vi "Find Running VIs.vi"(8 "error in":errorcluster, 10 "Find Sub-VIs (T)":bool=TRUE, 11 "Find Top-Level VIs (T)":bool=TRUE) -> (0 "error out":errorcluster, 1 "New VIs Found":string[][](array[string]), 2 "#VIs Found":i32, 3 "VIs Found":string[][](array[string]), 4 "#New VIs Found":i32)   [LabVIEW 2022 SP3, in "hse-misc.lvlib"]
doc: "____\nHAMPEL SOFTWARE ENGINEERING v3.8.0 (2023-12-18 14:41)"
uses:
  hse-misc.lvlib
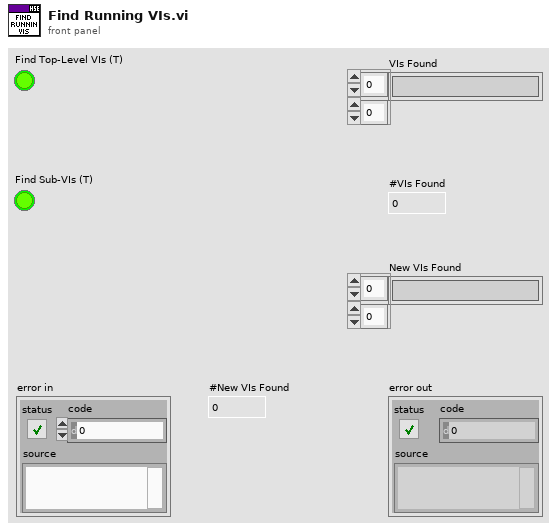
[diagram p1: front panel]
types:
  T1 = enum32{"Bad", "Idle", "Run top level", "Running"}
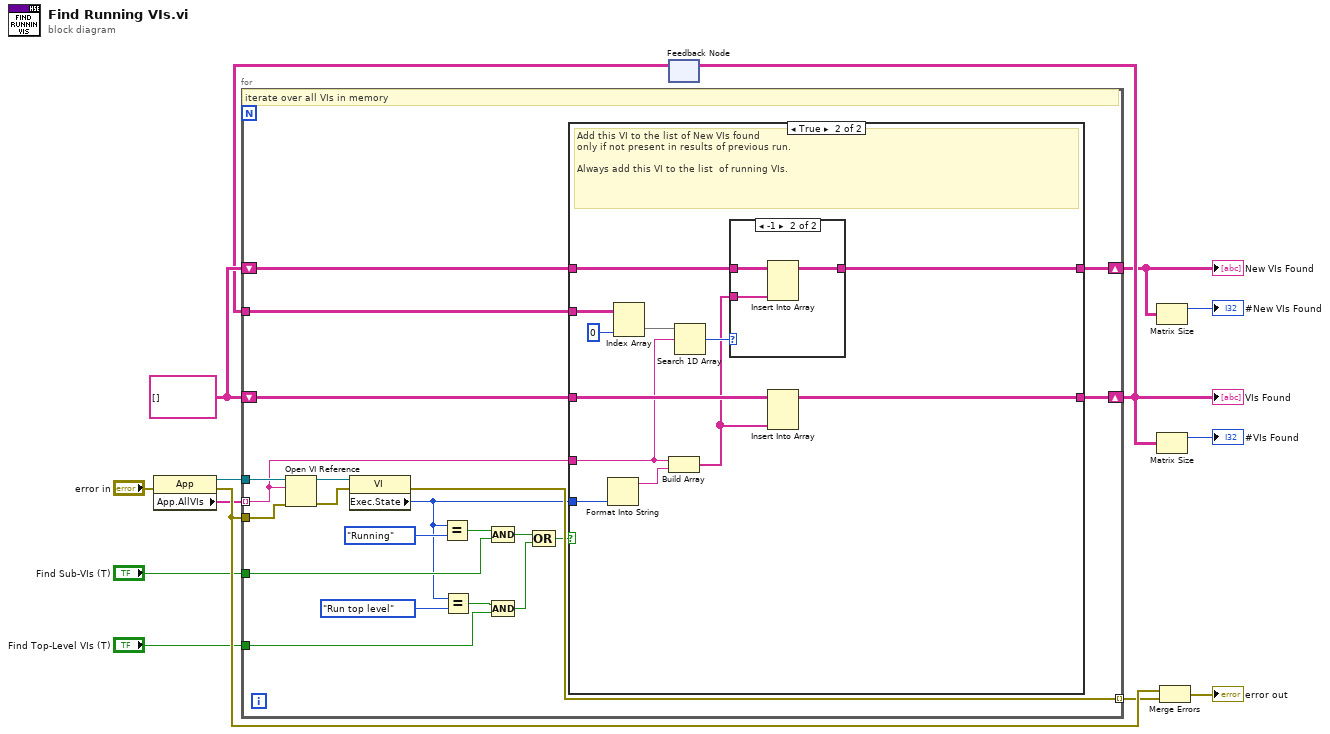
[diagram p0: block diagram]
diagram:
  w5 = string[][] []
  n1 = property class="App"(error in="error in") -> (reference out=w10:refnum<vi>, error out=w12:errorcluster, "App.AllVIs"=w11:string[])  [unwired: 1 in]
  n2 = feedback #1() -> (w3:string[][])  [unwired: 1 in]
  n3 = for {
    tunnel: w11 -> [w20] mode=indexing
    tunnel: w10 -> [w32]
    tunnel: w12 -> [w35]
    tunnel: "Find Top-Level VIs (T)" -> [w26]
    tunnel: "Find Sub-VIs (T)" -> [w25]
    shift-right: [w18] -> w4
    shift-left: w5 -> [w19]
    tunnel: [w33] -> w6 mode=indexing
    shift-right: [w16] -> w1
    shift-left: w5 -> [w15]
    tunnel: w3 -> [w17]
    # "iterate over all VIs in memory"
    n4 = Open VI Reference(application reference (local)=w32, vi path=w20, error in (no error)=w35) -> (vi reference=w31:refnum<vi>, error out=w34:errorcluster)  [unwired: 3 in]
    n5 = property class="VI"(reference=w31, error in=w34) -> (error out=w33:errorcluster, "Exec.State"=w21:T1)  [unwired: 1 out]
    n6 = Equal?(x=w21, y=T1."Running" ("Execution:State")) -> (x = y?=w28:bool)
    n7 = Equal?(x=w21, y=T1."Run top level" ("Execution:State")) -> (x = y?=w27:bool)
    n8 = Compound Arithmetic op=AND(w28, w25) -> (w24:bool)
    n9 = Compound Arithmetic op=AND(w27, w26) -> (w23:bool)
    n10 = Compound Arithmetic op=OR(w24, w23) -> (w22:bool)
    n11 = case shown="True" w22 {
      tunnel: w21 -> [_ w49]
      tunnel: w20 -> [_ w42]
      tunnel: w19 -> [w36 w47]
      tunnel: [w36 w46] -> w18
      tunnel: w17 -> [_ w45]
      tunnel: [w37 w40] -> w16
      tunnel: w15 -> [w37 w39]
      frame False {
      }
      frame True {
        # "Add this VI to the list of New VIs found\nonly if not present in results of previous run.\n\nAlways add this VI to the list  of running VIs."
        n12 = Format Into String(w49) -> (resulting string=w48:string)  [unwired: 3 in, 1 out]
        n13 = Index Array(array=w45, index (col)=0 ("disabled index (col)")) -> (element=w43:string[])  [unwired: 1 in]
        n14 = Build Array(w42, w48) -> (w38:string[])
        n15 = Search 1D Array(1D array=w43, element=w42) -> (index of element=w41:i32)  [unwired: 1 in]
        n16 = case shown="-1" w41 {
          tunnel: [w50 w52] -> w40
          tunnel: w39 -> [w50 w53]
          tunnel: w38 -> [_ w51]
          frame 0, Default {
          }
          frame -1 {
            n17 = Insert Into Array(array=w53, new element=w51) -> (w52:string[][])  [unwired: 2 in]
          }
        }
        n18 = Insert Into Array(array=w47, new element=w38) -> (w46:string[][])  [unwired: 2 in]
      }
    }
  }
  "VIs Found" <- w4
  "New VIs Found" <- w1
  n19 = feedback-in #1(w4) -> ()
  n20 = Matrix Size(0:w1) -> (1:→"#New VIs Found":i32)  [unwired: 1 out]
  n21 = Matrix Size(0:w4) -> (1:→"#VIs Found":i32)  [unwired: 1 out]
  n22 = Merge Errors(w12, w6) -> (→"error out":errorcluster)
